vi "Timed Loop Reset DUPE.vi"(8 "Bool Current State":bool, 9 "Bool Set":bool, 10 "Trigger Time(mS)":u32=1000, 11 "Last Event mS":u32) -> (0 "Bool Output":bool, 2 "Elapsed mS":u32, 3 "Last Event mS 2":u32)   [LabVIEW 2021]
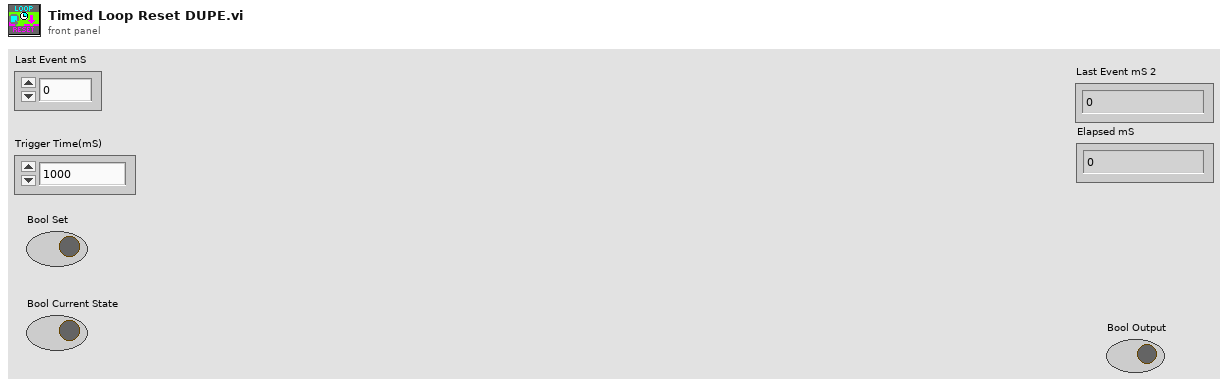
[diagram p1: front panel]
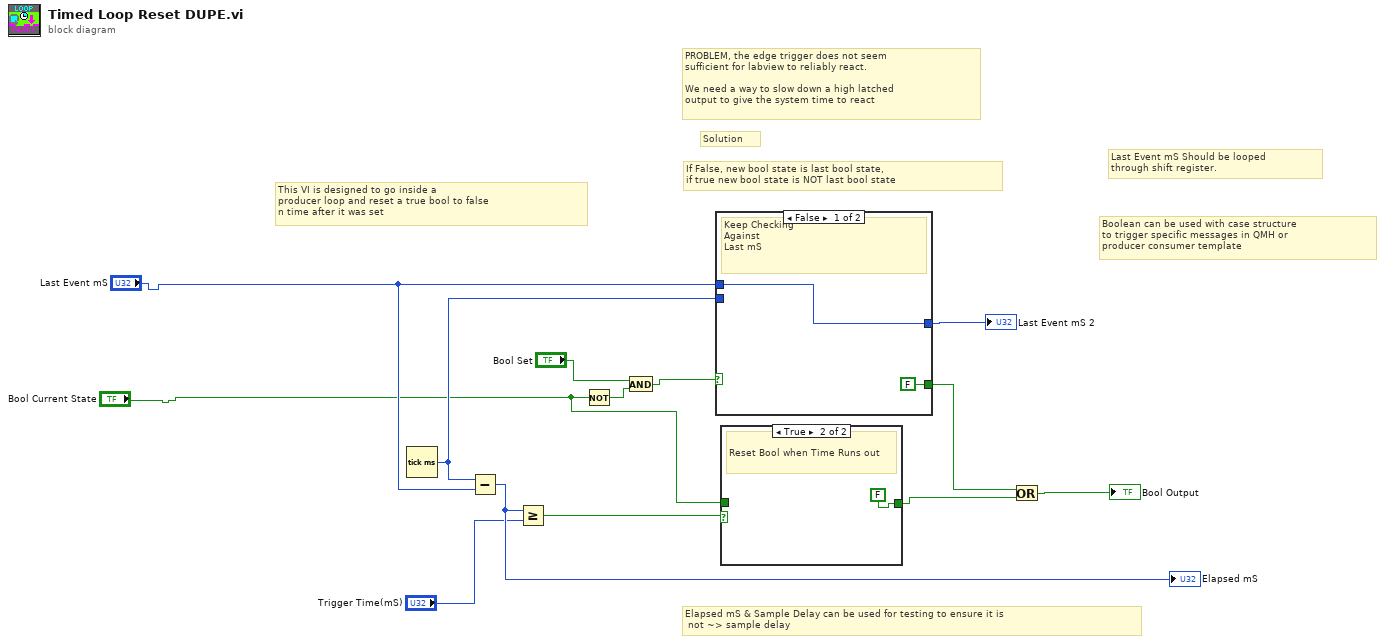
[diagram p0: block diagram]
diagram:
  # "Solution"
  # "If False, new bool state is last bool state,\nif true new bool state is NOT last bool state"
  # "PROBLEM, the edge trigger does not seem \nsufficient for labview to reliably react.\n\nWe need a way to slow down a high latched \noutput to give the system time to react"
  # "Elapsed mS & Sample Delay can be used for testing to ensure it is\n not ~> sample delay"
  # "Boolean can be used with case structure\nto trigger specific messages in QMH or \nproducer consumer template"
  # "This VI is designed to go inside a\nproducer loop and reset a true bool to false\nn time after it was set"
  # "Last Event mS Should be looped\nthrough shift register."
  n1 = Tick Count (ms)() -> (millisecond timer value=w12:u32)
  n2 = Subtract(x=w12, y="Last Event mS") -> (x-y=w13:u32)
  "Elapsed mS" <- w13
  n3 = Greater Or Equal?(x=w13, y="Trigger Time(mS)") -> (x >= y?=w10:bool)
  n4 = Not(x="Bool Current State") -> (.not. x?=w8:bool)
  n5 = And(x="Bool Set", y=w8) -> (x .and. y?=w7:bool)
  n6 = case shown="False" w7 {
    selector: w7 -> [_ w16]
    tunnel: [w15 w17] -> w3
    tunnel: w12 -> [_ w17]
    tunnel: "Last Event mS" -> [w15 _]
    tunnel: [FALSE w16] -> w6
    frame False {
      # "Keep Checking\nAgainst\nLast mS"
    }
    frame True {
      # "Save the \ncurrent mS"
    }
  }
  "Last Event mS 2" <- w3
  n7 = case shown="True" w10 {
    tunnel: "Bool Current State" -> [w18 _]
    tunnel: [w18 FALSE] -> w5
    frame False {
      # "Keep Checking\nAgainst\nLast mS"
    }
    frame True {
      # "Reset Bool when Time Runs out"
    }
  }
  n8 = Or(x=w6, y=w5) -> (x .or. y?=→"Bool Output":bool)
